vi "Receive test sting.vi"() -> ()   [LabVIEW 2012]
panel:
  out "Blinky":bool
  out "bytes?":bool
  out "return count":u32
  out "String Received":string
  in  "stop":bool
  in  "VISA resource name":refnum<visa-resource-name>="COM6"
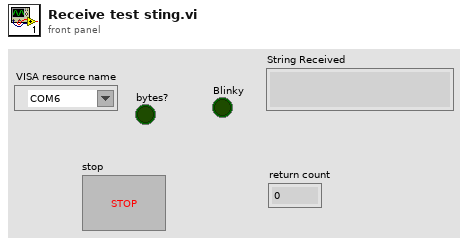
[diagram p1: front panel]
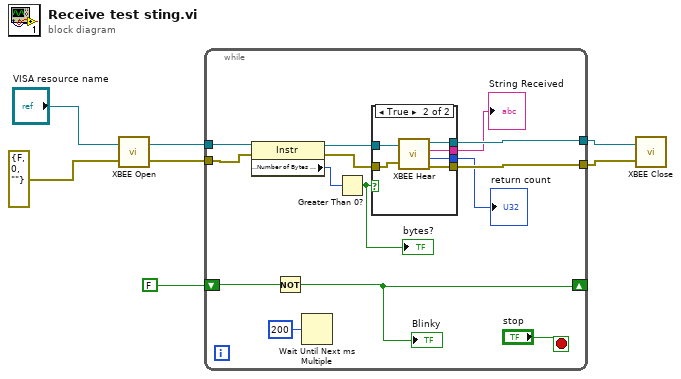
[diagram p0: block diagram]
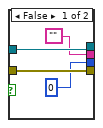
[diagram p2: hidden frame]
diagram:
  n1 = call "XBEE Open.vi"("error in"=errorcluster {"status"=FALSE, "code"=0, "source"=""}, "VISA resource name"="VISA resource name") -> ("error out"=w4:errorcluster, "VISA resource name out"=w5:refnum<visa-resource-name>)
  n2 = while {
    tunnel: w5 -> [w16]
    tunnel: w4 -> [w15]
    tunnel: [w20] -> w3
    tunnel: [w19] -> w2
    shift-right: [w8] -> _
    shift-left: FALSE -> [w9]
    stop <- "stop" stop-if-true
    n3 = property class="Instr"(reference=w16, error in=w15) -> (reference out=w13:refnum<visa-resource-name>, error out=w12:errorcluster, "Serial Settings:Number of Bytes at Serial Port"=w14:u32)
    n4 = Not(x=w9) -> (.not. x?=w8:bool)
    "Blinky" <- w8
    n5 = Wait Until Next ms Multiple(millisecond multiple=u32 200) -> ()  [unwired: 1 out]
    n6 = Greater Than 0?(x=w14) -> (x > 0?=w11:bool)
    "bytes?" <- w11
    n7 = case shown="True" w11 {
      tunnel: [w25 w31] -> w20
      tunnel: [w24 w30] -> w19
      tunnel: ["" w29] -> w18
      tunnel: [u32 0 ("return count") w28] -> w17
      tunnel: w13 -> [w25 w27]
      tunnel: w12 -> [w24 w26]
      frame False {
      }
      frame True {
        n8 = call "XBEE Hear.vi"("VISA resource name"=w27, "error in (no error)"=w26) -> ("VISA resource name out"=w31:refnum<visa-resource-name>, "String Received"=w29:string, "return count"=w28:u32, "error out"=w30:errorcluster)
      }
    }
    "String Received" <- w18
    "return count" <- w17
  }
  n9 = call "XBEE Close.vi"("error in (no error)"=w2, "VISA resource name"=w3) -> ()
